vi "OpenNetworkStreamWriter.vi"(7 "writer buffer size":i32, 8 "error in (no error)":errorcluster, 9 "reader url":string, 10 "writer name":string, 11 "NetworkStreamWriter in":refnum<class "NetworkStreamWriter.lvclass">) -> (0 "error out":errorcluster, 2 "Writer Endpoint":refnum<k21>, 3 "NetworkStreamWriter out":refnum<class "NetworkStreamWriter.lvclass">)   [LabVIEW 2011, in "NetworkStreamWriter.lvclass"]
doc: "Opens a network stream writer endpoint. This VI persistently tries to open the connection until it is successful or the e-stop is triggered."
uses:
  NetworkStreamWriter.lvclass
  Shared/message.ctl
  NetworkStreamWriter.lvclass/NetworkStreamWriter.ctl
  2-Think/2 Globals/2 Global.vi
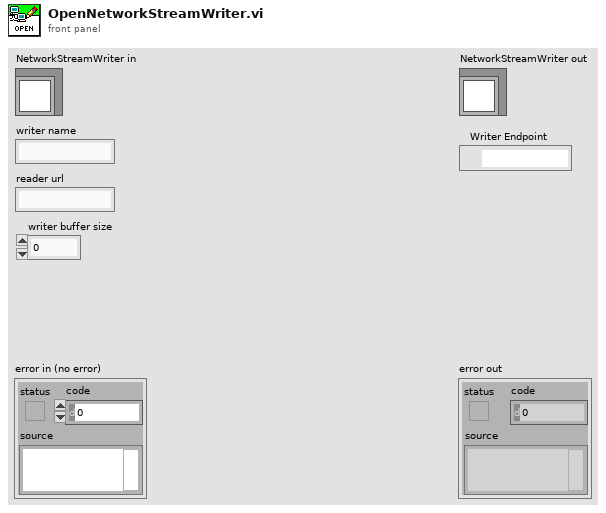
[diagram p1: front panel]
types:
  T1 = typedef "message.ctl" = cluster{"Data":variant, "Time since start (s)":dbl}
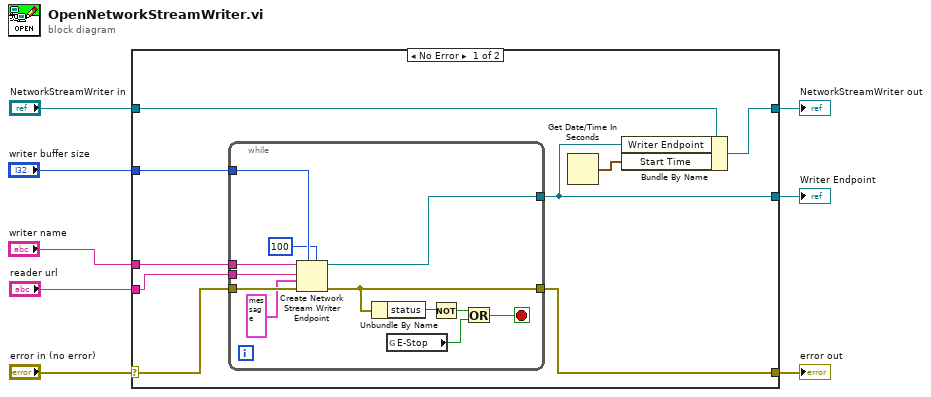
[diagram p0: block diagram]
diagram:
  n1 = case shown="No Error" "error in (no error)" {
    selector: "error in (no error)" -> [w17 w31]
    tunnel: [w15 w31] -> w7
    tunnel: [w13 w30] -> w5
    tunnel: "NetworkStreamWriter in" -> [w14 w30]
    tunnel: "writer buffer size" -> [w16 _]
    tunnel: "writer name" -> [w12 _]
    tunnel: "reader url" -> [w11 _]
    tunnel: [w10 _] -> w1
    frame No Error {
      n2 = while {
        tunnel: w17 -> [w29]
        tunnel: w16 -> [w28]
        tunnel: [w23] -> w15
        tunnel: w12 -> [w27]
        tunnel: w11 -> [w26]
        tunnel: [w19] -> w10
        stop <- w20 stop-if-true
        n3 = Create Network Stream Writer Endpoint(5:100 ("timeout in ms (-1)"), 7:w28, 8:w29, 9:T1 {"Data"=variant, "Time since start (s)"=0.0} ("variant"), 10:w26, 11:w27) -> (0:w23:errorcluster, 3:w19:refnum<k21>)
        n4 = Unbundle By Name(w23) -> ("status"=w22:bool)
        n5 = global read "2 Global.vi" "E-Stop"() -> (w18:bool)
        n6 = Not(x=w22) -> (.not. x?=w21:bool)
        n7 = Or(x=w21, y=w18) -> (x .or. y?=w20:bool)
      }
      n8 = Get Date/Time In Seconds() -> (seconds since 1Jan1904=w9:timestamp)
      n9 = Bundle By Name(cluster=w14, "Writer Endpoint"=w10, "Start Time"=w9) -> (w13:refnum<class "NetworkStreamWriter.lvclass">)
    }
    frame Error {
    }
  }
  "error out" <- w7
  "NetworkStreamWriter out" <- w5
  "Writer Endpoint" <- w1
